vi "TrajConstraint_GetMaxVelocity.vi"(7 "TrajjectoryConstraintType":T4, 8 "Velocity":dbl, 9 "Curvature":dbl, 10 "Pose":T1={"TRANSLATION"={"X"=0.0, "Y"=0.0}, "ROTATION"={"VALUE"=0.0, "COS"=1.0, "SIN"=0.0}} {"ROTATION"."SIN" format="%13.4f"; "ROTATION"."COS" format="%13.4f"; "ROTATION"."VALUE" format="%13.4f"; "TRANSLATION"."Y" format="%14.3f"; "TRANSLATION"."X" format="%14.3f"}, 11 "Trajectory Constraint":variant) -> (0 "error out":errorcluster, 3 "AbsMaxVelocity":dbl)   [LabVIEW 2019, in "Trajectory_Library.lvlib"]
doc: "Adds and enables a centripital acceleration constraint to ensure that the rotating capability of the robot is not exceeded.\n\nParameters:\n - MaxCentAccel - The maximum centripetal acceleration (meters/sec^2)\n - InTrajectoryConfig - The trajectory configuration data structure\n\nReturns:\n - OutTrajectoryConfig - Modified trajectory configuration data structure\n modified to conain them."
uses:
  Trajectory_Library.lvlib
  Enum/TRAJ_CONSTRAINT_TYPES_ENUM.ctl
  TypeDef/POSE2D.ctl
  TypeDef/TRANSLATION2D.ctl
  TypeDef/ROTATION2D.ctl
  TypeDef/TRAJ_CONSTRAINT_DIIF_DRIVE_KINEMATICS.ctl
  TypeDef/DIFF_DRIVE_KINEMATICS.ctl
  TypeDef/TRAJ_CONSTRAINT_DIIF_DRIVE_VOLTAGE.ctl
  TypeDef/SIMPLE_MOTOR_FF.ctl
  TypeDef/TRAJ_CONSTRAINT_CENTRIPETAL_ACCEL.ctl
  TypeDef/TRAJ_CONSTRAINT_MECA_DRIVE_KINEMATICS.ctl
  TypeDef/MECA_DRIVE_KINEMATICS.ctl
  <vilib>/Analysis/Matrix/Datatypes/RealMatrix.ctl
  TypeDef/TRAJ_CONSTRAINT_SWERVE_DRIVE_KINEMATICS.ctl
  TypeDef/SWERVE_DRIVE_KINEMATICS.ctl
  TypeDef/TRAJ_CONSTRAINT_MAX_VELOCITY.ctl
  <vilib>/Analysis/Matrix/NI_Matrix.lvlib
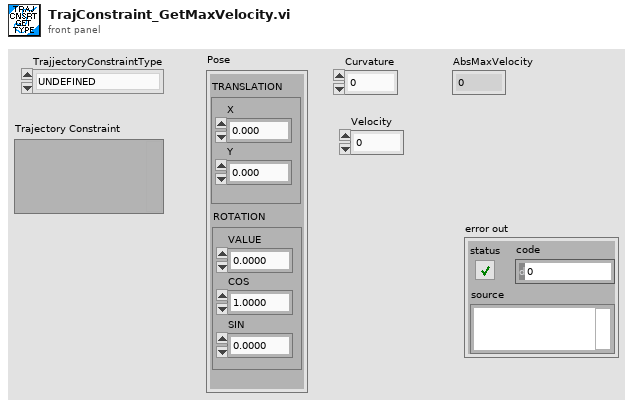
[diagram p1: front panel]
types:
  T1 = typedef "Trajectory_Library.lvlib/POSE2D.ctl" = cluster{"TRANSLATION":T2, "ROTATION":T3}
  T2 = typedef "Trajectory_Library.lvlib/TRANSLATION2D.ctl" = cluster{"X":dbl, "Y":dbl}
  T3 = typedef "Trajectory_Library.lvlib/ROTATION2D.ctl" = cluster{"VALUE":dbl, "COS":dbl, "SIN":dbl}
  T4 = typedef "Trajectory_Library.lvlib/TRAJ_CONSTRAINT_TYPES_ENUM.ctl" = enum16{"UNDEFINED", "DIFF DRIVE KINEMATICS", "DIFF DRIVE VOLTAGE", "CENTRIPITAL ACCEL", "MECA DRIVE KINEMATICS", "SWERVE DRIVE KINEMATICS", "MAXIMUM VELOCITY", "ELLIPTICAL REGION", "RECTANGULAR REGION"}
  T5 = typedef "Trajectory_Library.lvlib/TRAJ_CONSTRAINT_DIIF_DRIVE_KINEMATICS.ctl" = cluster{"Max Speed (M/S)":dbl, "DIFF_DRIVE_KINEMATICS":T6, "Max Accel (M/S2)":dbl}
  T6 = typedef "Trajectory_Library.lvlib/DIFF_DRIVE_KINEMATICS.ctl" = cluster{"TrackWidth_Meters":dbl}
  T7 = typedef "Trajectory_Library.lvlib/TRAJ_CONSTRAINT_DIIF_DRIVE_VOLTAGE.ctl" = cluster{"Max Voltage":dbl, "DIFF_DRIVE_KINEMATICS":T6, "SIMPLE_MOTOR_FF":T8}
  T8 = typedef "Trajectory_Library.lvlib/SIMPLE_MOTOR_FF.ctl" = cluster{"Ks":dbl, "Kv":dbl, "Ka":dbl}
  T9 = typedef "Trajectory_Library.lvlib/TRAJ_CONSTRAINT_CENTRIPETAL_ACCEL.ctl" = cluster{"Max Cent Accel":dbl}
  T10 = typedef "Trajectory_Library.lvlib/TRAJ_CONSTRAINT_MECA_DRIVE_KINEMATICS.ctl" = cluster{"Max Speed (M/S)":dbl, "MECA_DRIVE_KINEMATICS":T11}
  T11 = typedef "Trajectory_Library.lvlib/MECA_DRIVE_KINEMATICS.ctl" = cluster{"FrontLeft":T2, "FrontRight":T2, "RearLeft":T2, "RearRight":T2, "InverseKinematics":T12, "ForwardKinematics":T12, "PrevCoR":T2}
  T12 = typedef "NI_Matrix.lvlib/RealMatrix.ctl" = dbl[][]
  T13 = typedef "Trajectory_Library.lvlib/TRAJ_CONSTRAINT_SWERVE_DRIVE_KINEMATICS.ctl" = cluster{"Max Speed (M/S)":dbl, "SwerveKinematics":T14}
  T14 = typedef "Trajectory_Library.lvlib/SWERVE_DRIVE_KINEMATICS.ctl" = cluster{"NumModules":i32, "InverseKinematics":T12, "ForwardKinematics":T12, "Modules":T2[], "PrevCoR":T2}
  T15 = typedef "Trajectory_Library.lvlib/TRAJ_CONSTRAINT_MAX_VELOCITY.ctl" = cluster{"Max Velocity":dbl, "IM UNIQUE":bool}
  T16 = typedef "Trajectory_Library.lvlib/TRAJ_CONSTRAINT_MINMAX.ctl" = cluster{"minAccel":dbl, "maxAccel":dbl}
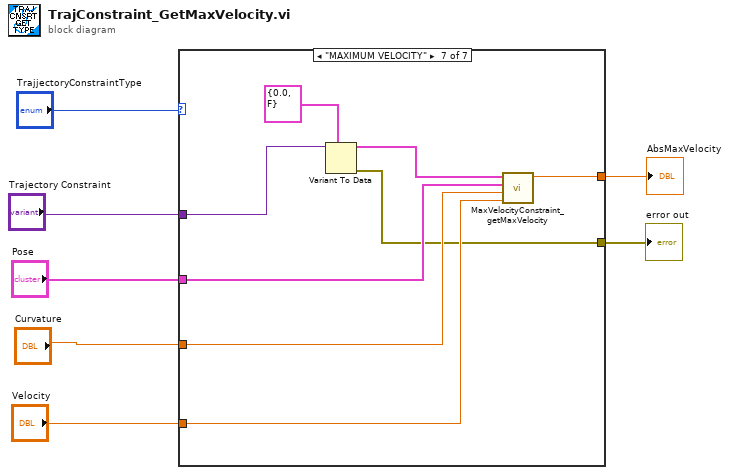
[diagram p0: block diagram]
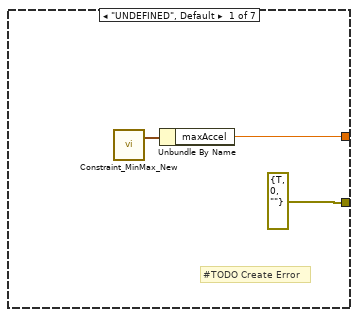
[diagram p2: hidden frame]
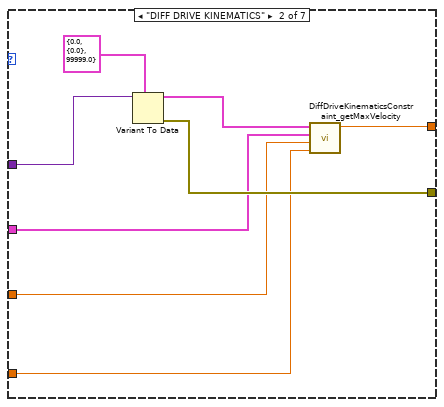
[diagram p3: hidden frame]
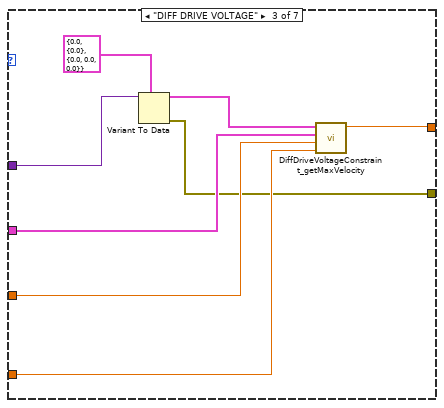
[diagram p4: hidden frame]
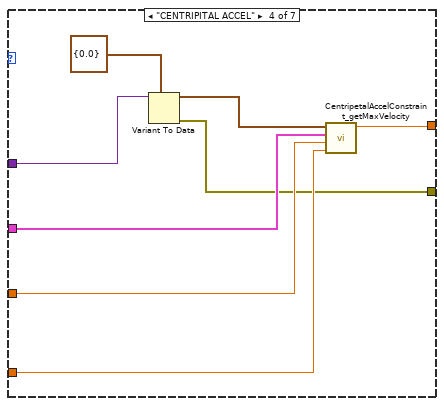
[diagram p5: hidden frame]
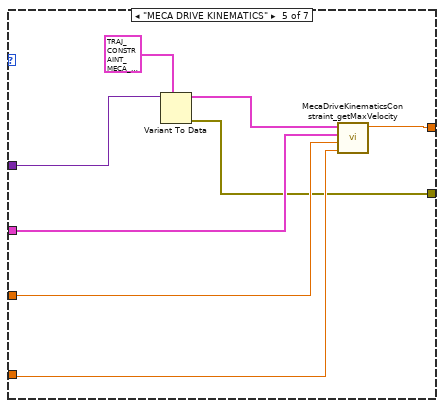
[diagram p6: hidden frame]
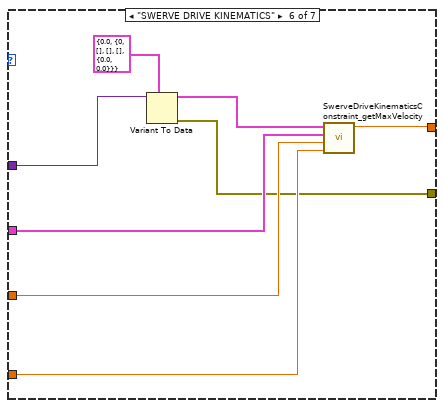
[diagram p7: hidden frame]
diagram:
  n1 = case shown="\"MAXIMUM VELOCITY\"" "TrajjectoryConstraintType" {
    tunnel: [w9 w11 w19 w32 w40 w48 w55] -> w7
    tunnel: "Trajectory Constraint" -> [_ w17 w21 w27 w35 w43 w56]
    tunnel: [errorcluster {"status"=TRUE, "code"=0, "source"=""} ("error out") w15 w20 w28 w36 w44 w51] -> w6
    tunnel: "Pose" -> [_ w14 w24 w31 w39 w47 w54]
    tunnel: "Curvature" -> [_ w13 w23 w30 w38 w46 w53]
    tunnel: "Velocity" -> [_ w12 w22 w29 w37 w45 w52]
    frame "UNDEFINED", Default {
      # "#TODO Create Error"
      n2 = call "Constraint_MinMax_New.vi"() -> ("TRAJ_CONSTAINT_MIN_MAX"=w10:T16)  [unwired: 11 in]
      n3 = Unbundle By Name(w10) -> ("maxAccel"=w9:dbl)
    }
    frame "DIFF DRIVE KINEMATICS" {
      n4 = Variant To Data(type=T5 {"Max Speed (M/S)"=0.0, "DIFF_DRIVE_KINEMATICS"={"TrackWidth_Meters"=0.0}, "Max Accel (M/S2)"=99999.0} ("DIFF_DRIVE_KINE_CONSTRAINT"), Variant=w17) -> (data=w16:T5, error out=w15:errorcluster)  [unwired: 1 in]
      n5 = call "DiffDriveKinematicsConstraint_getMaxVelocity.vi"("Velocity"=w12, "Curvature"=w13, "statePose"=w14, "DIFF_DRIVE_KINE_CONSTRAINT"=w16) -> ("absMaxVelocity"=w11:dbl)  [unwired: 7 in]
    }
    frame "DIFF DRIVE VOLTAGE" {
      n6 = Variant To Data(type=T7 {"Max Voltage"=0.0, "DIFF_DRIVE_KINEMATICS"={"TrackWidth_Meters"=0.0}, "SIMPLE_MOTOR_FF"={"Ks"=0.0, "Kv"=0.0, "Ka"=0.0}} ("DIFF_DRIVE_VOLTAGE_CONSTRAINT"), Variant=w21) -> (data=w25:T7, error out=w20:errorcluster)  [unwired: 1 in]
      n7 = call "DiffDriveVoltageConstraint_getMaxVelocity.vi"("Velocity"=w22, "Curvature"=w23, "statePose"=w24, "DIFF_DRIVE_VOLTAGE_CONSTRAINT"=w25) -> ("absMaxVelocity"=w19:dbl)  [unwired: 7 in]
    }
    frame "CENTRIPITAL ACCEL" {
      n8 = Variant To Data(type=T9 {"Max Cent Accel"=0.0} ("CENTRIPETAL_ACCEL_CONSTRAINT"), Variant=w27) -> (data=w33:T9, error out=w28:errorcluster)  [unwired: 1 in]
      n9 = call "CentripetalAccelConstraint_getMaxVelocity.vi"("Velocity"=w29, "Curvature"=w30, "statePose"=w31, "CENTRIPETAL_ACCEL_CONSTRAINT"=w33) -> ("absMaxVelocity"=w32:dbl)  [unwired: 7 in]
    }
    frame "MECA DRIVE KINEMATICS" {
      n10 = Variant To Data(type=T10 {"Max Speed (M/S)"=0.0, "MECA_DRIVE_KINEMATICS"={"FrontLeft"={"X"=0.0, "Y"=0.0}, "FrontRight"={"X"=0.0, "Y"=0.0}, "RearLeft"={"X"=0.0, "Y"=0.0}, "RearRight"={"X"=0.0, "Y"=0.0}, "InverseKinematics"=[[0.0, 1.0, -1.0, 0.0], [0.0, 1.0, 1.0, 0.0], [0.0, 1.0, 1.0, 0.0], [0.0, 1.0, -1.0, 0.0]], "ForwardKinematics"=[[0.0, 1.0, -1.0, 0.0], [0.0, 1.0, 1.0, 0.0], [0.0, 1.0, 1.0, 0.0], [0.0, 1.0, -1.0, 0.0]], "PrevCoR"={"X"=0.0, "Y"=0.0}}} ("MECANUM_DRIVE_KINE_CONSTRAINT"), Variant=w35) -> (data=w41:T10, error out=w36:errorcluster)  [unwired: 1 in]
      n11 = call "MecaDriveKinematicsConstraint_getMaxVelocity.vi"("Velocity"=w37, "Curvature"=w38, "statePose"=w39, "MECANUM_DRIVE_KINE_CONSTRAINT"=w41) -> ("absMaxVelocity"=w40:dbl)  [unwired: 7 in]
    }
    frame "SWERVE DRIVE KINEMATICS" {
      n12 = Variant To Data(type=T13 {"Max Speed (M/S)"=0.0, "SwerveKinematics"={"NumModules"=0, "InverseKinematics"=[], "ForwardKinematics"=[], "Modules"=[], "PrevCoR"={"X"=0.0, "Y"=0.0}}} ("SWERVE_DRIVE_KINE_CONSTRAINT"), Variant=w43) -> (data=w49:T13, error out=w44:errorcluster)  [unwired: 1 in]
      n13 = call "SwerveDriveKinematicsConstraint_getMaxVelocity.vi"("Velocity"=w45, "Curvature"=w46, "statePose"=w47, "SWERVE_DRIVE_KINE_CONSTRAINT"=w49) -> ("absMaxVelocity"=w48:dbl)  [unwired: 7 in]
    }
    frame "MAXIMUM VELOCITY" {
      n14 = Variant To Data(type=T15 {"Max Velocity"=0.0, "IM UNIQUE"=FALSE} ("MAX_VELOCITY_CONSTRAINT"), Variant=w56) -> (data=w57:T15, error out=w51:errorcluster)  [unwired: 1 in]
      n15 = call "MaxVelocityConstraint_getMaxVelocity.vi"("Velocity"=w52, "Curvature"=w53, "statePose"=w54, "MAX_VELOCITY_CONSTRAINT"=w57) -> ("absMaxVelocity"=w55:dbl)  [unwired: 7 in]
    }
  }
  "AbsMaxVelocity" <- w7
  "error out" <- w6
